vi "HackedComm.vi"(8 "error in (no error)":errorcluster, 11 "Data":T1) -> (0 "error out":errorcluster, 3 "Communication":T2)   [LabVIEW 2020]
uses:
  RestAPI.ctl
  JSON_Formats.vi
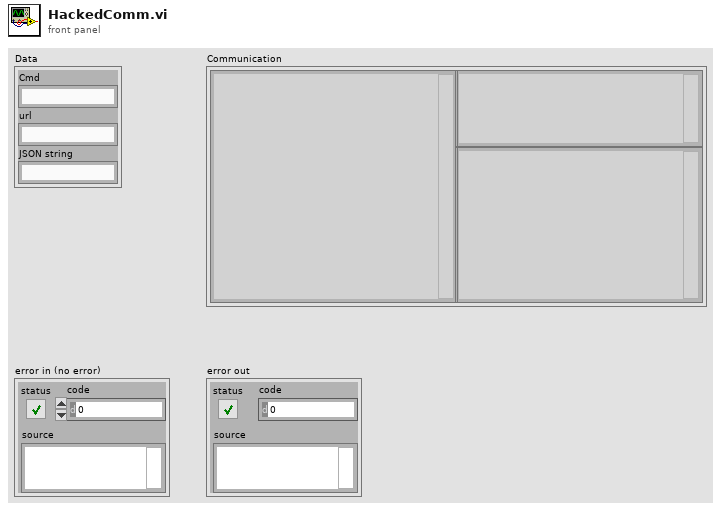
[diagram p1: front panel]
types:
  T1 = cluster{"Cmd":string, "url":string, "JSON string":string}
  T2 = typedef "RestAPI.ctl" = cluster{"headers 2":string, "headers":string, "body":string}
  T3 = cluster{"cmd":string, "path":string, "http ver":string}
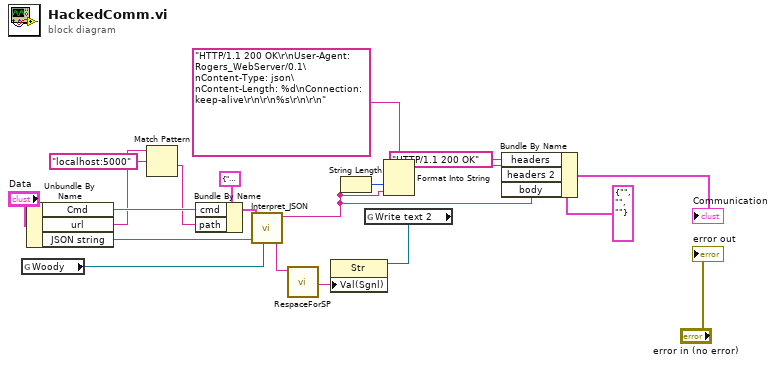
[diagram p0: block diagram]
diagram:
  n1 = global read "JSON_Formats.vi" "Woody"() -> (w12:refnum<vi>)
  n2 = Unbundle By Name("Data") -> ("Cmd"=w14:string, "url"=w3:string, "JSON string"=w16:string)
  n3 = Match Pattern(string=w3, regular expression="localhost:5000") -> (after substring=w2:string)  [unwired: 1 in, 3 out]
  n4 = Bundle By Name(cluster=T3 {"cmd"="GET", "path"="/state", "http ver"="HTTP/1.1"} ("path"), "cmd"=w14, "path"=w2) -> (w13:T3)
  n5 = call "Interpret_JSON.vi"("Server VI"=w12, "payload"=w16, "Command"=w13) -> ("Send to Server"=w18:string, "Read from Server"=w5:string)  [unwired: 6 in, 1 out]
  n6 = call "RespaceForSP.vi"("Code"=w18) -> ("Cleaned for SPIKE"=w19:string)  [unwired: 10 in]
  n7 = String Length(string=w5) -> (length=w10:i32)
  n8 = global read "JSON_Formats.vi" "Write text 2"() -> (w11:refnum<vi>)
  n9 = property on="Property Node" class="Str"(reference=w11, "Val(Sgnl)"=w19) -> ()  [unwired: 1 in, 2 out]
  n10 = Format Into String(format string="HTTP/1.1 200 OK\r\nUser-Agent: Rogers_WebServer/0.1\nContent-Type: json\nContent-Length: %d\nConnection: keep-alive\r\n\r\n%s\r\n\r\n" ("regular expression"), w10, w5) -> (resulting string=w7:string)  [unwired: 2 in, 1 out]
  n11 = Bundle By Name(cluster=T2 {"headers 2"="", "headers"="", "body"=""} ("Communication"), "headers"="HTTP/1.1 200 OK", "headers 2"=w7, "body"=w5) -> (→"Communication":T2)
  "error out" <- "error in (no error)"
